vi "Agilent WriteConfigFile.vi"(9 "Dispositivos":string[][](table)=[["Armario1", "CH  1", "SO2", "50000", "ppm", "0.00"], ["Armario1", "CH  2", "NO", "2500", "ppm", "0.00"], ["Armario1", "CH  3", "CO", "10000", "ppm", "0.00"], ["Armario1", "CH  4", "CO2", "25.0", "%", "0.00"], ["Armario1", "CH  5", "O2 ", "25.0", "%", "0.00"], ["Armario1", "CH  6", "", "", "", "0.00"], ["Armario1", "CH  7", "", "", "", "0.00"], ["Armario1", "CH  8", "", "", "", "0.00"], ["Armario2", "CH  9", "CH4", "30.0", "%", "0.00"], ["Armario2", "CH 10", "CO", "100.0", "%", "0.00"], ["Armario2", "CH 11", "H2", "60.0", "%", "0.00"], ["Armario2", "CH 12", "CO", "20.0", "%", "0.00"], ["Armario2", "CH 13", "CO2", "100.0", "%", "0.00"], ["Armario2", "CH 14", "CH4", "20.0", "%", "0.00"], ["Armario2", "CH 15", "", "", "", "0.00"], ["Armario2", "CH 16", "", "", "", "0.00"], ["Armario3", "CH 17", "", "", "", "0.00"], ["Armario3", "CH 18", "", "", "", "0.00"], ["Armario3", "CH 19", "H2", "100.0", "%", "0.00"], ["Armario3", "CH 20", "CO", "100.0", "%", "0.00"], ["Armario3", "CH 21", "CO2", "100.0", "%", "0.00"], ["Armario3", "CH 22", "", "", "", "0.00"], ["Armario3", "CH 23", "", "", "", "0.00"], ["Armario3", "CH 24", "", "", "", "0.00"], ["Armario4", "CH 25", "O2", "60.0", "%", "0.00"], ["Armario4", "CH 26", "CO", "50.0", "%", "0.00"], ["Armario4", "CH 27", "CO2", "100.0", "%", "0.00"], ["Armario4", "CH 28", "CH4", "50.0", "%", "0.00"], ["Armario4", "CH 29", "H2", "50.0", "%", "0.00"], ["Armario4", "CH 30", "", "", "", "0.00"], ["Armario4", "CH 31", "", "", "", "0.00"], ["Armario4", "CH 32", "", "", "", "0.00"], ["Armario5", "CH 33", "O2", "25.0", "%", "0.00"], ["Armario5", "CH 34", "CO2", "30.0", "%", "0.00"], ["Armario5", "CH 35", "CO", "3.0", "%", "0.00"], ["Armario5", "CH 36", "O2", "25.0", "%", "0.00"], ["Armario5", "CH 37", "CO2", "100.0", "%", "0.00"], ["Armario5", "CH 38", "CO", "5.0", "%", "0.00"], ["Armario5", "CH 39", "SO2", "5000", "ppm", "0.00"], ["Armario5", "CH 40", "", "", "", "0.00"]] caption="Tabla de medidores de gases") -> (0 "Error Out":errorcluster)   [LabVIEW 2017]
doc: "Illustrates how to create and write a configuration settings file.\n\nInstructions:\nEnter values in the controls on the front panel then click on the Run Arrow.\nTo read the file, run Read Configuration Settings File.vi located in the file\\config.llb."
uses:
  <vilib>/Utility/config.llb/Write Key (String).vi
  <vilib>/Utility/config.llb/NI_LVConfig.lvlib
panel:
  in  "Error In":errorcluster
  out "configuration file path":path
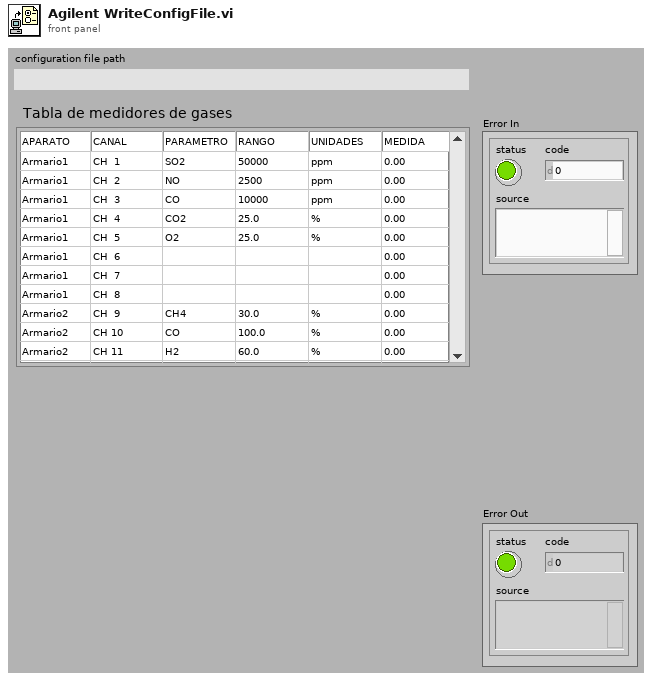
[diagram p1: front panel]
types:
  T1 = typedef "NI_LVConfig.lvlib/Config Data RefNum.ctl" = refnum<k1>
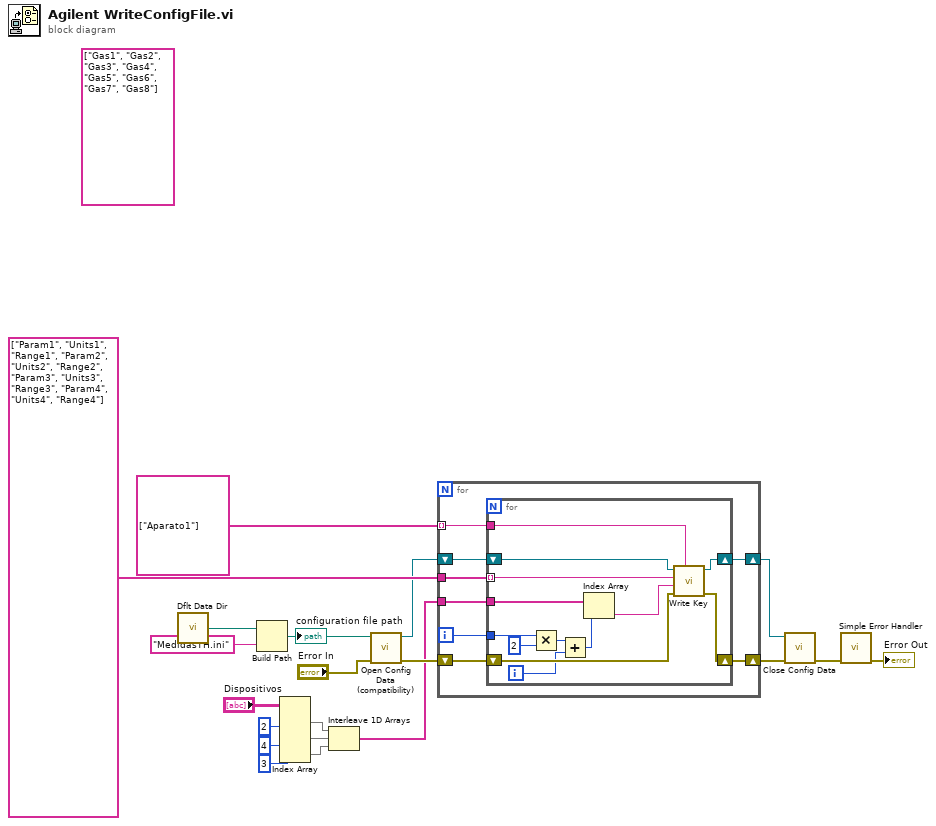
[diagram p0: block diagram]
diagram:
  (unwired) string[] ["Gas1", "Gas2", "Gas3", "Gas4", "Gas5", "Gas6", "Gas7", "Gas8"]
  n1 = call <vilib>:"Dflt Data Dir.vi"() -> ("App:Default Data Directory"=w18:path)
  n2 = Build Path(base path=w18, name or relative path="MedidasTH.ini") -> (appended path=w17:path)
  "configuration file path" <- w17
  n3 = Index Array(array="Dispositivos", index (col) #1=2 ("disabled index (col)"), index (col) #2=4 ("index (col)"), index (col) #3=3 ("index (col)")) -> (element #1=w3:string[], element #2=w5:string[], element #3=w4:string[])  [unwired: 3 in]
  n4 = Interleave 1D Arrays(w3, w5, w4) -> (w2:string[])
  n5 = call <vilib>:"Open Config Data (compatibility).vi"("error in (no error)"="Error In", "configuration file path"=w17) -> ("error out"=w10:errorcluster, "refnum"=w13:T1)  [unwired: 7 in, 1 out]
  n6 = for {
    shift-right: [w26] -> w12
    shift-left: w10 -> [w27]
    tunnel: string[] ["Aparato1"] -> [w24] mode=indexing
    tunnel: string[] ["Param1", "Units1", "Range1", "Param2", "Units2", "Range2", "Param3", "Units3", "Range3", "Param4", "Units4", "Range4"] -> [w25]
    shift-right: [w23] -> w11
    shift-left: w13 -> [w28]
    tunnel: w2 -> [w22]
    i -> [w21]
    n7 = for {
      shift-right: [w38] -> w26
      shift-left: w27 -> [w39]
      tunnel: w25 -> [w40] mode=indexing
      tunnel: w24 -> [w41]
      shift-right: [w36] -> w23
      shift-left: w28 -> [w37]
      tunnel: w22 -> [w35]
      tunnel: w21 -> [w34]
      i -> [w29]
      n8 = Multiply(x=w34, y=2) -> (x*y=w32:i32)
      n9 = Add(x=w32, y=w29) -> (x+y=w30:i32)
      n10 = Index Array(array=w35, index=w30) -> (element=w31:string)
      n11 = call-poly <vilib>:"Write Key.vi"("section"=w41, "error in (no error)"=w39, "value"=w31, "key"=w40, "refnum"=w37) -> ("error out"=w38:errorcluster, "refnum out"=w36:T1)  [unwired: 4 in, 1 out]
    }
  }
  n12 = call <vilib>:"Close Config Data.vi"("error in (no error)"=w12, "refnum"=w11) -> ("error out"=w20:errorcluster)  [unwired: 8 in, 1 out]
  n13 = call <vilib>:"Simple Error Handler.vi"("error in (no error)"=w20) -> ("error out"=→"Error Out":errorcluster)  [unwired: 4 in, 4 out]
